vi "Read Busy Flag and Address.vi"(6 "chip select (1st chip)":enum16{"1st chip", "2nd chip"}(ring), 8 "error in (no error)":errorcluster, 11 "LCD in":u32) -> (0 "error out":errorcluster, 1 "address":u8=97 format="%.0x", 2 "busy flag":bool, 3 "LCD out":u32)   [LabVIEW 2015, in "HD44780 FPGA.lvlib"]
doc: "Checks whether a character LCD device is busy and reads the current address."
uses:
  <vilib>/EmbeddedDisplay/Hitachi HD44780/FPGA/HD44780 FPGA.lvlib
  <vilib>/EmbeddedDisplay/Hitachi HD44780/Common/HD44780 Common.lvlib
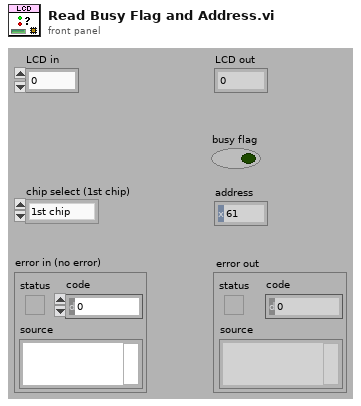
[diagram p1: front panel]
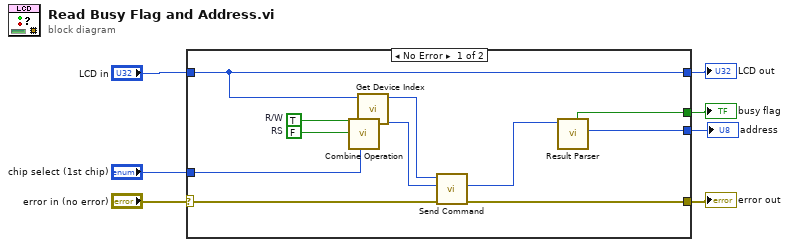
[diagram p0: block diagram]
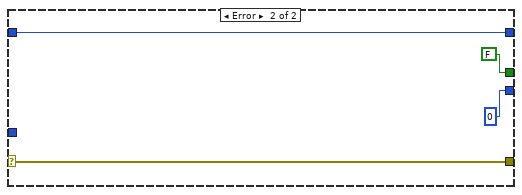
[diagram p2: hidden frame]
diagram:
  n1 = case shown="No Error" "error in (no error)" {
    selector: "error in (no error)" -> [w15 w22]
    tunnel: [w14 w22] -> w6
    tunnel: "chip select (1st chip)" -> [w16 _]
    tunnel: "LCD in" -> [w9 w21]
    tunnel: [w9 w21] -> w3
    tunnel: [w13 FALSE] -> w2
    tunnel: [w12 u8 0] -> w1
    frame No Error {
      w17 = TRUE  # R/W
      w18 = FALSE  # RS
      n2 = call <vilib>:"Combine Operation.vi"("chip select  (1st chip)"=w16, "RS"=w18, "R/W"=w17) -> ("output"=w11:u32)  [unwired: 8 in]
      n3 = call <vilib>:"Get Device Index.vi"("LCD in"=w9) -> ("device index"=w8:i8)  [unwired: 10 in]
      n4 = call <vilib>:"Send Command.vi"("error in (no error)"=w15, "operation"=w11, "device index"=w8) -> ("error out"=w14:errorcluster, "Result"=w10:u32)  [unwired: 6 in, 1 out]
      n5 = call <vilib>:"Result Parser.vi"("operation"=w10) -> ("address"=w12:u8, "busy flag"=w13:bool)  [unwired: 8 in, 1 out]
    }
    frame Error {
    }
  }
  "error out" <- w6
  "LCD out" <- w3
  "busy flag" <- w2
  "address" <- w1
